vi "Create Refnum And Add To Cluster.vi"(8 "error in":errorcluster, 9 "Owning Cluster in":refnum<vi>, 10 "Ctl Refnum":refnum<vi>) -> (0 "error out":errorcluster, 1 "Owning Cluster out":refnum<vi>, 2 "Created RefNum":refnum<vi>)   [LabVIEW 2021, in "_Msg.lvlib"]
uses:
  <vilib>/Utility/miscctls.llb/LVPositionTypeDef.ctl
  _Msg.lvlib
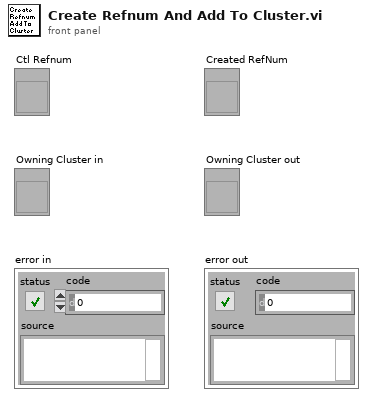
[diagram p1: front panel]
types:
  T1 = typedef "LVPositionTypeDef.ctl" = cluster{"Left":i32, "Top":i32}
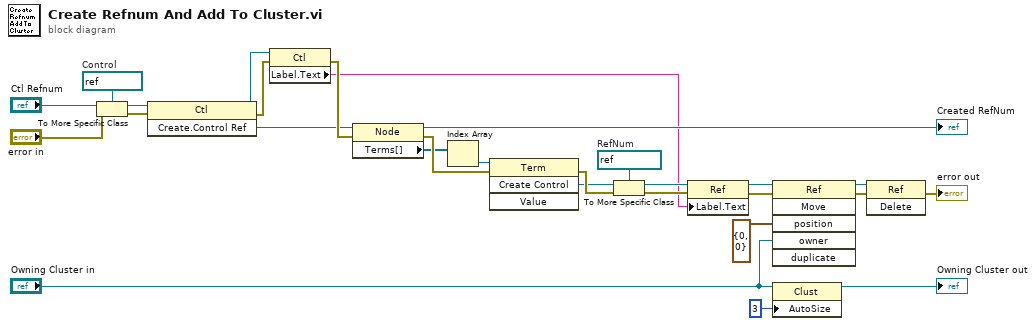
[diagram p0: block diagram]
diagram:
  w12 = refnum<vi> refnum  # RefNum
  w15 = refnum<vi> refnum  # Control
  n1 = To More Specific Class(target class=w15, reference="Ctl Refnum", error in="error in") -> (specific class reference=w10:refnum<vi>, error out=w22:errorcluster)
  n2 = invoke class="Ctl" method="Create.Control Ref"(reference=w10, error in=w22) -> (reference out=w8:refnum<vi>, error out=w21:errorcluster, "Create Control Ref"=w9:refnum<vi>)  [unwired: 1 in]
  n3 = property class="Ctl"(reference=w8, error in=w21) -> (error out=w17:errorcluster, "Label.Text"=w4:string)  [unwired: 1 out]
  n4 = property class="Node"(reference=w9, error in=w17) -> (reference out=→"Created RefNum":refnum<vi>, error out=w20:errorcluster, "Terms[]"=w14:refnum<vi>[])
  n5 = Index Array(array=w14) -> (element=w13:refnum<vi>)  [unwired: 1 in]
  n6 = invoke class="Term" method="Create Control"(reference=w13, error in=w20) -> (error out=w2:errorcluster, "Create Control"=w1:refnum<vi>)  [unwired: 2 in, 2 out]
  n7 = To More Specific Class(target class=w12, reference=w1, error in=w2) -> (specific class reference=w7:refnum<vi>, error out=w19:errorcluster)
  n8 = property class="Ref"(reference=w7, error in=w19, "Label.Text"=w4) -> (reference out=w6:refnum<vi>, error out=w16:errorcluster)
  n9 = invoke class="Ref" method="Move"(reference=w6, error in=w16, "position"=T1 {"Left"=0, "Top"=0}, "owner"="Owning Cluster in") -> (reference out=w5:refnum<vi>, error out=w18:errorcluster)  [unwired: 2 in, 4 out]
  n10 = property class="Clust"(reference="Owning Cluster in", "AutoSize"=u32 3 ("Auto Sizing")) -> (reference out=→"Owning Cluster out":refnum<vi>)  [unwired: 1 in, 1 out]
  n11 = invoke class="Ref" method="Delete"(reference=w5, error in=w18) -> (error out=→"error out":errorcluster)  [unwired: 1 in, 2 out]
